vi "jMsg_StoreNameUpdate (create).vi"(8 "error in (no error)":errorcluster, 11 "Name":string) -> (0 "error out":errorcluster, 3 "jMsg_StoreNameUpdate":refnum<class "jMsg_StoreNameUpdate.lvclass">)   [LabVIEW 2020, in "jMsg_StoreNameUpdate.lvclass"]
doc: "This VI is used to create the jMsg\n\n\nJSMA Message Wizard 0.2.0.5\nRob Humfeld - Jet Engineering\nCopyright (c) 2020, Jet Engineering"
uses:
  jMsg_StoreNameUpdate.lvclass
  C:/Program Files/National Instruments/LabVIEW 2020/user.lib/JET Engineering/JSMA/Libraries/jMsg Class/jMsg.lvclass
  <userlib>/JET Engineering/JSMA/Libraries/jMsg Class/jMsg.lvclass/jMsg.ctl
  jMsg_StoreNameUpdate.lvclass/jMsg_StoreNameUpdate.ctl
  <userlib>/JET Engineering/JSMA/Libraries/Shared/JSMA_GetClassName.vi
  <vilib>/Utility/LVClass/Get LV Class Path.vi
  <userlib>/JET Engineering/JSMA/Libraries/jMsg Class/jMsg.lvclass
panel:
  in  "jMsg_StoreNameUpdate":refnum<class "jMsg_StoreNameUpdate.lvclass">
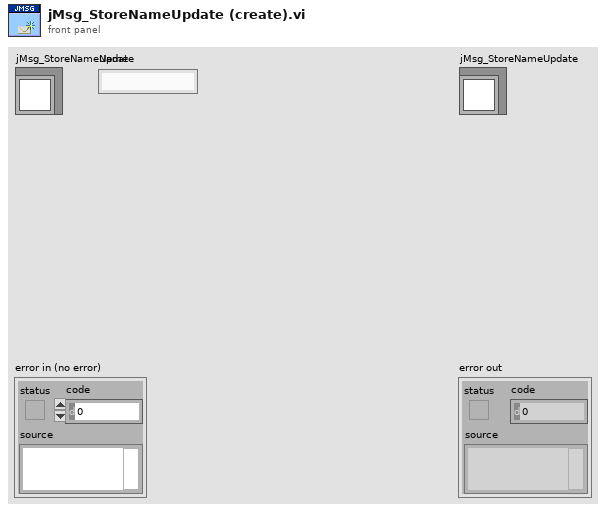
[diagram p1: front panel]
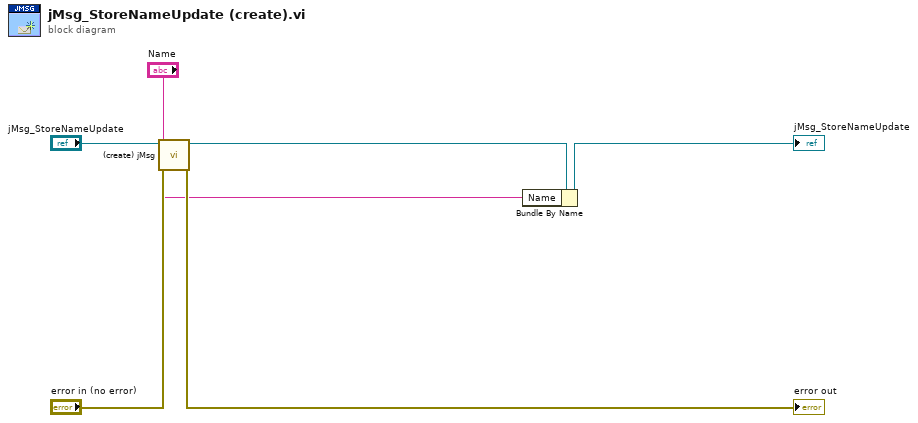
[diagram p0: block diagram]
diagram:
  n1 = call <userlib>:"(create) jMsg.vi"("error in (no error)"="error in (no error)", "jMsg in"="jMsg_StoreNameUpdate") -> ("error out"=→"error out":errorcluster, "jMsg out"=w2:refnum<class "jMsg_StoreNameUpdate.lvclass">)  [unwired: 8 in]
  n2 = Bundle By Name(cluster=w2, "Name"="Name") -> (→"jMsg_StoreNameUpdate":refnum<class "jMsg_StoreNameUpdate.lvclass">)
